vi "TEST-JSON-RPC.vi"() -> ()   [LabVIEW 2019]
uses:
  typedefs/Response--Cluster.ctl
  typedefs/Request--Cluster.ctl
  typedefs/Notification Object--Cluster.ctl
  typedefs/Error Object--Cluster.ctl
  JSON-RPC.lvclass
panel:
  out "Array 2":string[](array[string])
  out "Array":dbl[][](array[numeric])
  in  "Numeric":i32=3
  in  "Notification":bool
  in  "Request.method":string
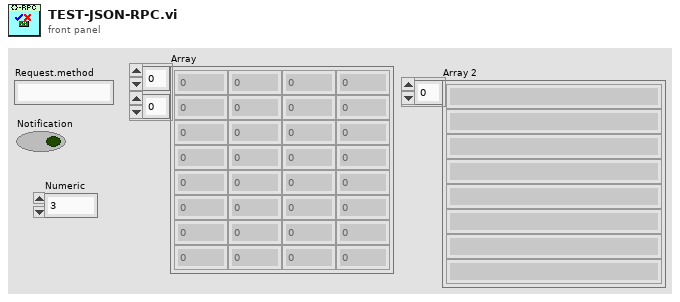
[diagram p1: front panel]
types:
  T1 = typedef "JSON-RPC.lvclass/Error Object--Cluster.ctl" = cluster{"code":i32, "message":string, "data":variant}
  T2 = typedef "JSON-RPC.lvclass/Notification Object--Cluster.ctl" = cluster{"method":string, "params":variant}
  T3 = typedef "JSON-RPC.lvclass/Request--Cluster.ctl" = cluster{"method":string, "params":variant, "Notification?":bool}
  T4 = typedef "JSON-RPC.lvclass/Response--Cluster.ctl" = cluster{"jasonrpc":string, "result":variant, "error":variant}
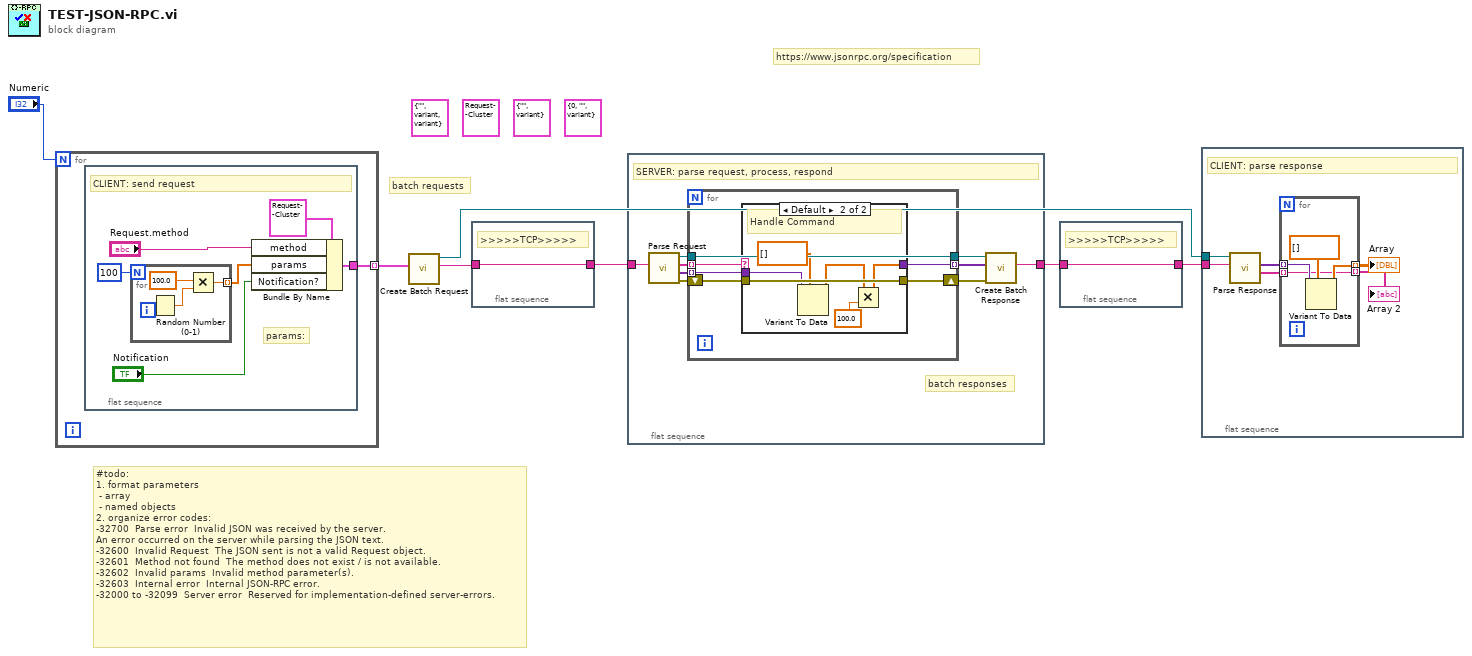
[diagram p0: block diagram]
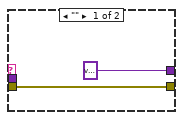
[diagram p2: hidden frame]
diagram:
  (unwired) T1 {"code"=0, "message"="", "data"=variant} ("Error")
  (unwired) T2 {"method"="", "params"=variant} ("notification")
  (unwired) T3 {"method"="", "params"=variant, "Notification?"=FALSE} ("request")
  (unwired) T4 {"jasonrpc"="", "result"=variant, "error"=variant} ("response")
  # "#todo:\n1. format parameters\n - array\n - named objects\n2. organize error codes:\n-32700 \tParse error \tInvalid JSON was received by the server.\nAn error occurred on the server while parsing the JSON text.\n-32600 \tInvalid Request \tThe JSON sent is not a valid Request object.\n-32601 \tMethod not found \tThe method does not exist / is not available.\n-32602 \tInvalid params \tInvalid method parameter(s).\n-32603 \tInternal error \tInternal JSON-RPC error.\n-32000 to -32099 \tServer error \tReserved for implementation-defined server-errors."
  # "batch requests"
  # "https://www.jsonrpc.org/specification"
  n1 = for {
    N: "Numeric" -> [_]
    tunnel: [w8] -> w5 mode=indexing
    n2 = flat-sequence {
      tunnel: [w10] -> w8
      frame #0 {
        # "params:"
        # "CLIENT: send request"
        n3 = for {
          N: 100 -> [_]
          tunnel: [w17] -> w9 mode=indexing
          n4 = Random Number (0-1)() -> (number: 0 to 1=w15:dbl)
          n5 = Multiply(x=100.0, y=w15) -> (x*y=w17:dbl)
        }
        n6 = Bundle By Name(cluster=T3 {"method"="", "params"=variant, "Notification?"=FALSE} ("request"), "method"="Request.method", "params"=w9, "Notification?"="Notification") -> (w10:T3)
      }
    }
  }
  n7 = call "Create Batch Request.vi"("Requests"=w5) -> ("Request"=w4:string, "JSON-RPC out"=w2:refnum<class "JSON-RPC.lvclass">)  [unwired: 8 in, 1 out]
  n8 = flat-sequence {
    tunnel: w4 -> [w18]
    tunnel: [w18] -> w7
    frame #0 {
      # ">>>>>TCP>>>>>"
    }
  }
  n9 = flat-sequence {
    tunnel: w7 -> [w27]
    tunnel: [w20] -> w1
    frame #0 {
      # "batch responses"
      # "SERVER: parse request, process, respond"
      n10 = call "Parse Request.vi"("JSON Request"=w27) -> ("error out"=w26:errorcluster, "Params"=w25:variant[], "Methods"=w24:string[], "JSON-RPC out"=w23:refnum<class "JSON-RPC.lvclass">)  [unwired: 7 in]
      n11 = for {
        tunnel: w25 -> [w32] mode=indexing
        tunnel: w24 -> [w31] mode=indexing
        tunnel: w23 -> [w28]
        tunnel: [w29] -> w19 mode=indexing
        shift-right: [w30] -> w22
        shift-left: w26 -> [w33]
        tunnel: [w28] -> w21
        n12 = case shown="Default" w31 {
          tunnel: w33 -> [w35 w41]
          tunnel: [w35 w41] -> w30
          tunnel: [variant ("Variant") w37] -> w29
          tunnel: w32 -> [_ w40]
          frame "" {
          }
          frame Default {
            # "Handle Command"
            n13 = Variant To Data(type=dbl[] [], Variant=w40) -> (data=w38:dbl[])  [unwired: 1 in, 1 out]
            n14 = Multiply(x=w38, y=100.0 ("x")) -> (x*y=w37:dbl[])
          }
        }
      }
      n15 = call "Create Batch Response.vi"("error in (no error)"=w22, "results"=w19, "JSON-RPC in"=w21) -> ("Response"=w20:string)  [unwired: 6 in, 2 out]
    }
  }
  n16 = flat-sequence {
    tunnel: w1 -> [w42]
    tunnel: [w42] -> w3
    frame #0 {
      # ">>>>>TCP>>>>>"
    }
  }
  n17 = flat-sequence {
    tunnel: w3 -> [w48]
    tunnel: w2 -> [w47]
    frame #0 {
      # "CLIENT: parse response"
      n18 = call "Parse Response.vi"("JSON Request"=w48, "JSON-RPC in"=w47) -> ("ids"=w45:string[], "Results"=w46:variant[])  [unwired: 6 in, 2 out]
      n19 = for {
        tunnel: w46 -> [w52] mode=indexing
        tunnel: w45 -> [w49] mode=indexing
        tunnel: [w50] -> w44 mode=indexing
        tunnel: [w49] -> w43 mode=indexing
        n20 = Variant To Data(type=dbl[] [], Variant=w52) -> (data=w50:dbl[])  [unwired: 1 in, 1 out]
      }
      "Array" <- w44
      "Array 2" <- w43
    }
  }
